vi "Rate_scan_standalone.vi"() -> ()   [LabVIEW 2019]
panel:
  out "Waveform Graph":dbl[][](graph)
  out "Errores":dbl
  out "Valor escrito":u16 format="%.0x"
  out "Iteraciones":i32
  out "Sumador":u64
  out "Canal":u64
  out "Amplitude":dbl
  out "LLTHx":dbl
  out "HLTHx":dbl
  out "WRITE OK":bool
  in  "stop":bool
  out "Valor leido":u16 format="%x"
  out "DAC\nTH3,TH4,TH5":u16 format="%x"
  out "DAC\nTH0,TH1,TH2":u16 format="%x"
  out "Scaler 1":u16
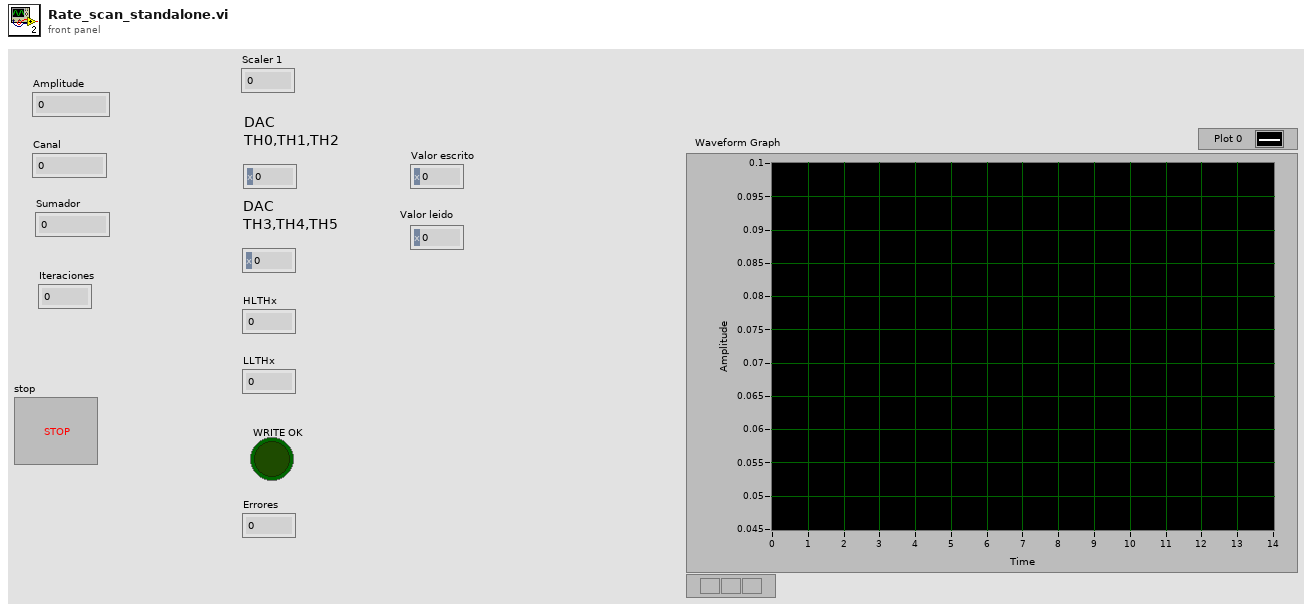
[diagram p1: front panel]
types:
  T1 = cluster{"Device Index":u32, "FT_FLAGS_OPENED":bool, "FT_FLAGS_HISPEED":bool, "Type":u32, "VID":u32, "PID":u32, "LocID":i32, "Serial Number":string, "Description":string, "FT_Handle":u32}
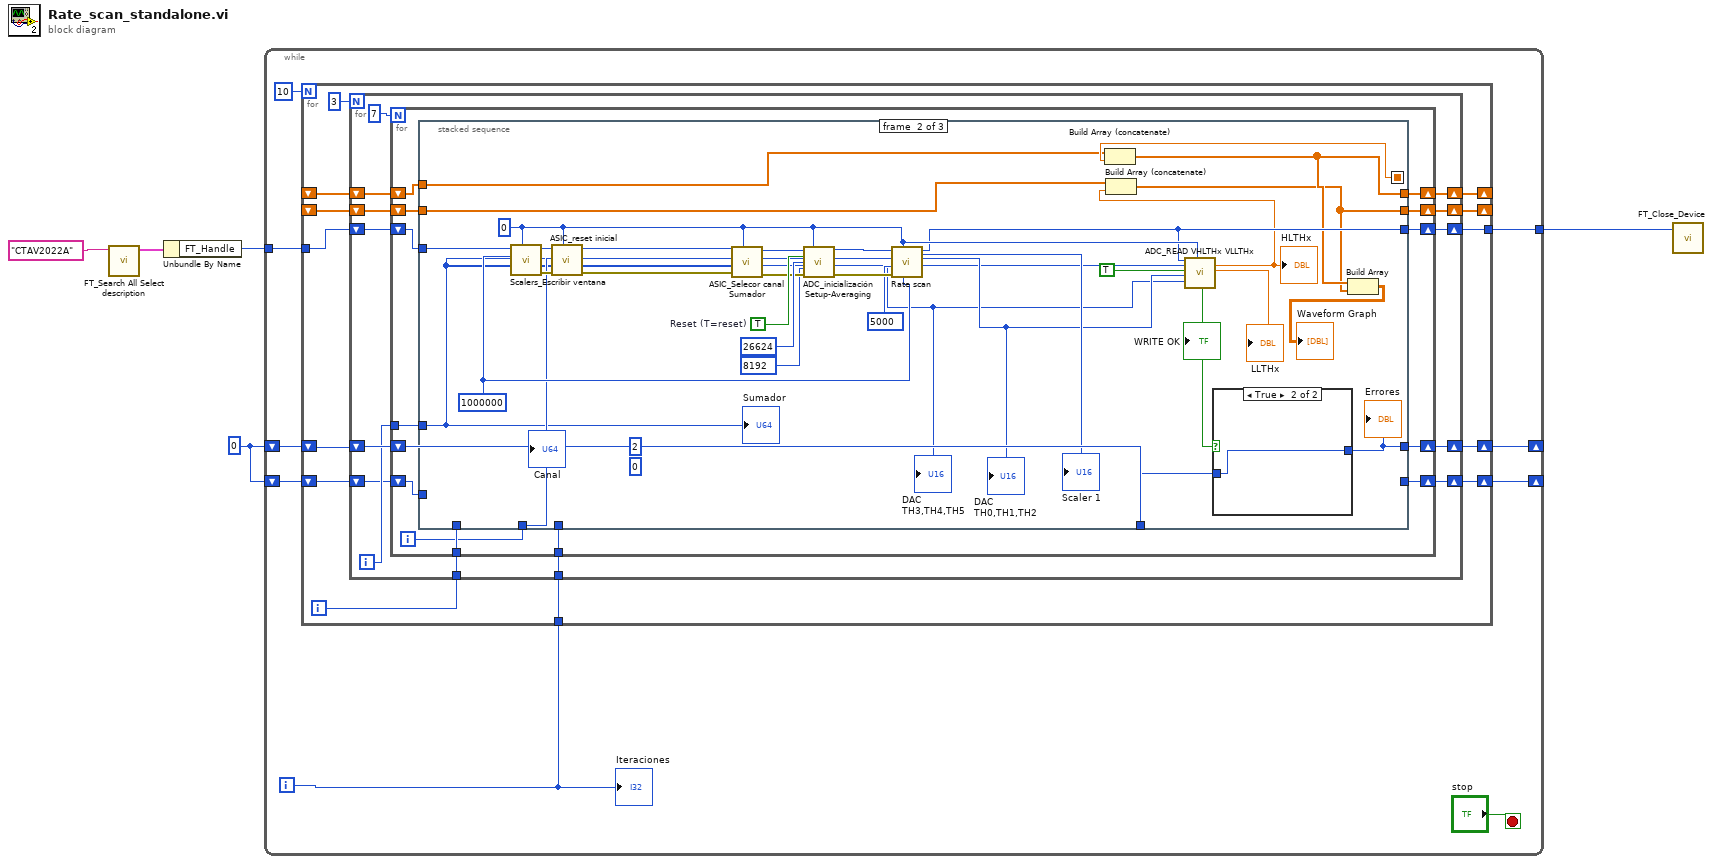
[diagram p0: block diagram]
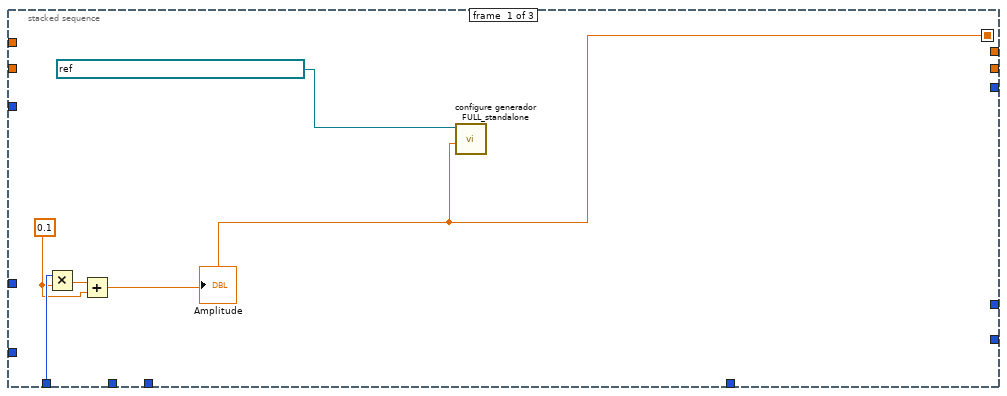
[diagram p2: hidden frame]
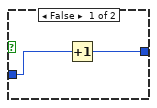
[diagram p3: hidden frame]
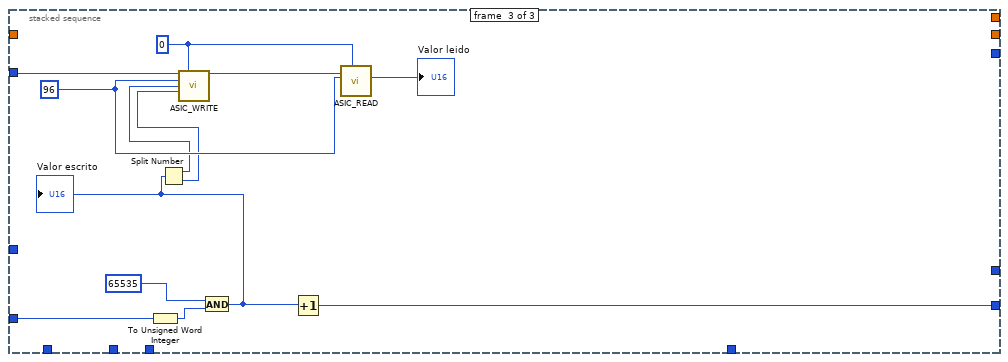
[diagram p4: hidden frame]
diagram:
  w1 = u64 0 ("lower bound (0)")
  n1 = call "FT_Search All Select description.vi"("CTA Test#"="CTAV2022A") -> ("Select Ft"=w5:T1)  [unwired: 8 in, 2 out]
  n2 = Unbundle By Name(w5) -> ("FT_Handle"=w3:u32)
  n3 = while {
    tunnel: w3 -> [w9]
    tunnel: [w10] -> w2
    shift-right: [w12] -> _
    shift-left: w1 -> [w11]
    shift-right: [w7] -> _
    shift-left: w1 -> [w6]
    i -> [w14]
    stop <- "stop" stop-if-true
    n4 = for {
      N: 10 -> [_]
      tunnel: w14 -> [w27]
      shift-right: [w26] -> w12
      shift-left: w11 -> [w25]
      tunnel: [w24] -> w10
      tunnel: w9 -> [w23]
      shift-right: [w20] -> w7
      shift-left: w6 -> [w19]
      shift-right: [w18] -> _
      shift-left: _ -> [w17]
      shift-right: [w16] -> _
      shift-left: _ -> [w15]
      i -> [w22]
      n5 = for {
        N: 3 -> [_]
        tunnel: w27 -> [w41]
        tunnel: w22 -> [w36]
        shift-right: [w40] -> w26
        shift-left: w25 -> [w39]
        shift-right: [w38] -> w24
        shift-left: w23 -> [w37]
        shift-right: [w33] -> w20
        shift-left: w19 -> [w32]
        shift-right: [w31] -> w18
        shift-left: w17 -> [w30]
        shift-right: [w29] -> w16
        shift-left: w15 -> [w28]
        i -> [w35]
        n6 = for {
          N: 7 -> [_]
          tunnel: w41 -> [w55]
          tunnel: w36 -> [w50]
          tunnel: w35 -> [w49]
          shift-right: [w54] -> w40
          shift-left: w39 -> [w53]
          shift-right: [w52] -> w38
          shift-left: w37 -> [w51]
          shift-right: [w47] -> w33
          shift-left: w32 -> [w46]
          shift-right: [w45] -> w31
          shift-left: w30 -> [w44]
          shift-right: [w43] -> w29
          shift-left: w28 -> [w42]
          i -> [w48]
          n7 = stacked-sequence {
            seq-local: [w56 _ _] -> [_ w68 _]
            tunnel: w51 -> [_ w79 w103]
            tunnel: w55 -> [_ _ _]
            tunnel: [_ w77 _] -> w52
            tunnel: [_ w71 _] -> w54
            tunnel: w53 -> [_ w70 _]
            tunnel: w50 -> [w59 _ _]
            tunnel: w49 -> [_ w61 _]
            tunnel: w48 -> [_ w69 _]
            tunnel: [_ _ w98] -> w47
            tunnel: w46 -> [_ _ w97]
            tunnel: [_ w64 _] -> w45
            tunnel: w44 -> [_ w67 _]
            tunnel: [_ w63 _] -> w43
            tunnel: w42 -> [_ w65 _]
            frame #0 {
              w57 = 0.1 ("y")
              n8 = Multiply(x=w59, y=w57) -> (x*y=w58:dbl)
              n9 = Add(x=w58, y=w57) -> (x+y=w56:dbl)
              "Amplitude" <- w56
              n10 = call "configure generador FULL_standalone.vi"("Amplitude (1.0 Vpp)"=w56, "VISA Key 81160A"=refnum<visa-resource-name> "USB0::0x0957::0x4108::MY51400682::INSTR") -> ()  [unwired: 7 in, 3 out]
            }
            frame #1 {
              (unwired) u64 2 ("upper bound (100)")
              (unwired) u64 0 ("lower bound (0)")
              w81 = u32 1000000 ("Ventana")
              w78 = u32 0 ("Espera acceso USB")
              w93 = TRUE  # Reset (T=reset)
              n11 = call "Scalers_Escribir ventana.vi"("Espera acceso USB"=w78, "Ventana"=w81, "ftHandle_in"=w79) -> ("error out"=w84:errorcluster, "ftHandle_out"=w85:u32)  [unwired: 7 in]
              n12 = call "ASIC_reset inicial.vi"("Espera acceso USB"=w78, "error in"=w84, "ftHandle_in"=w85) -> ("error out"=w83:errorcluster, "ftHandle_out"=w82:u32)  [unwired: 7 in]
              n13 = call "ASIC_Selecor canal Sumador.vi"("Espera acceso USB"=w78, "error in"=w83, "Sumador"=w61, "Canal"=w69, "ftHandle_in"=w82) -> ("error out"=w91:errorcluster, "ftHandle_out"=w90:u32)  [unwired: 4 in, 1 out]
              n14 = call "ADC_inicialización Setup-Averaging.vi"("ftHandle_in 2"=w90, "Espera acceso USB"=w78, "Reset (T=reset)"=w93, "Registro Setup (0x6800)"=u16 26624, "Registro Averaging (0x3200)"=u16 8192 ("Registro Setup (0x6800)"), "error in 2"=w91) -> ("ftHandle_out"=w88:u32, "error out"=w87:errorcluster)  [unwired: 8 in]
              n15 = call "Rate scan.vi"("T Ventana"=w81, "Espera acceso USB"=w78, "error in 2"=w87, "Valor buscado scalers (5000)"=u16 5000 ("Valor buscado scalers"), "Sumador"=w61, "ftHandle_in 2"=w88) -> ("DAC\nTH3,TH4,TH5"=w74:u16, "DAC\nTH0,TH1,TH2"=w75:u16, "ftHandle_out 2"=w77:u32, "Scaler 1"=→"Scaler 1":u16)  [unwired: 1 in, 1 out]
              "DAC\nTH0,TH1,TH2" <- w75
              "DAC\nTH3,TH4,TH5" <- w74
              n16 = Build Array (concatenate)(w67, w68) -> (w64:dbl[])
              n17 = call "ADC_READ VHLTHx VLLTHx.vi"("ftHandle_out 2"=w77, "Sumador"=w61, "referenciar"=TRUE, "ref DAC\nTH0,TH1,TH2"=w75, "ref DAC\nTH3,TH4,TH5"=w74, "Espera acceso FT"=w78) -> ("WRITE OK"=w72:bool, "HLTHx"=w66:dbl, "LLTHx"=→"LLTHx":dbl)  [unwired: 9 in, 2 out]
              "WRITE OK" <- w72
              "HLTHx" <- w66
              n18 = Build Array (concatenate)(w65, w66) -> (w63:dbl[])
              n19 = case shown="True" w72 {
                tunnel: [w95 w96] -> w71
                tunnel: w70 -> [w94 w96]
                frame False {
                  n20 = Increment(x=w94) -> (x+1=w95:u64)
                }
                frame True {
                }
              }
              "Errores" <- w71
              n21 = Build Array(w64, w63) -> (→"Waveform Graph":dbl[][])
              "Canal" <- w69
              "Sumador" <- w61
            }
            frame #2 {
              w107 = u8 96 ("Direccion Registro Asic")
              w108 = u32 0 ("Espera acceso USB")
              n22 = To Unsigned Word Integer(number=w97) -> (unsigned 16bit integer=w101:u16)
              n23 = And(x=u16 65535, y=w101) -> (x .and. y?=w99:u16)
              "Valor escrito" <- w99
              n24 = Split Number(x=w99) -> (hi(x)=w105:u8, lo(x)=w104:u8)
              n25 = call "ASIC_WRITE.vi"("ftHandle_in"=w103, "Espera acceso USB"=w108, "Direccion Registro Asic"=w107, "Byte Alto"=w105, "Byte Bajo"=w104) -> ("ftHandle_out"=w106:u32)  [unwired: 9 in, 1 out]
              n26 = Increment(x=w99) -> (x+1=w98:u16)
              n27 = call "ASIC_READ.vi"("Espera acceso USB"=w108, "Direccion Registro Asic"=w107, "ftHandle_in"=w106) -> ("Valor Asic"=→"Valor leido":u16)  [unwired: 6 in, 2 out]
            }
          }
        }
      }
    }
    "Iteraciones" <- w14
  }
  n28 = call "FT_Close_Device.vi"("Handle"=w2) -> ()  [unwired: 1 out]
